vi "Update device interface.vi"(8 "error in (no error)":errorcluster, 10 "Found Instruments":string[][](array[string]), 11 "PIC-Device in":refnum<class "PIC-Device.lvclass">) -> (0 "error out":errorcluster, 3 "PIC-Device out":refnum<class "PIC-Device.lvclass">)   [LabVIEW 2020, in "PIC-Device.lvclass"]
uses:
  PIC-Device.lvclass
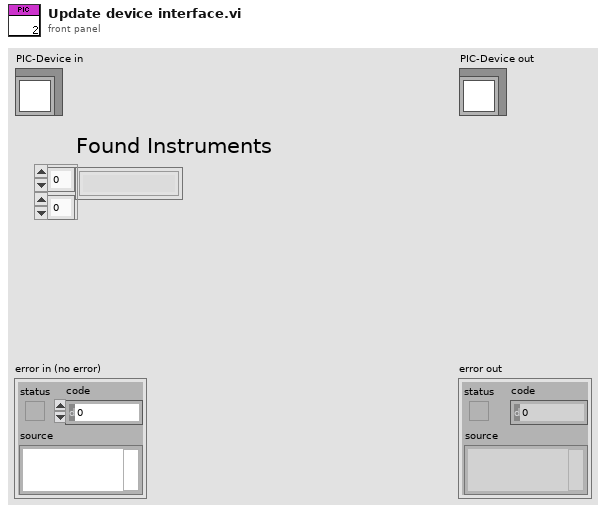
[diagram p1: front panel]
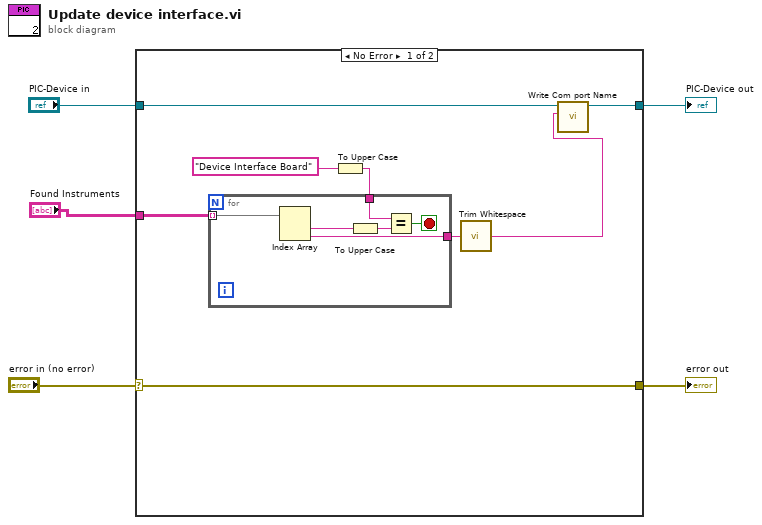
[diagram p0: block diagram]
diagram:
  n1 = case shown="No Error" "error in (no error)" {
    selector: "error in (no error)" -> [w13 w21]
    tunnel: [w13 w21] -> w4
    tunnel: [w11 w20] -> w3
    tunnel: "PIC-Device in" -> [w12 w20]
    tunnel: "Found Instruments" -> [w10 _]
    frame No Error {
      n2 = To Upper Case(1:"Device Interface Board") -> (0:w8:string)
      n3 = for {
        tunnel: w10 -> [w19] mode=indexing
        tunnel: w8 -> [w17]
        tunnel: [w15] -> w7
        stop <- w14 stop-if-true
        n4 = Index Array(array=w19) -> (element #1=w18:string, element #2=w15:string)  [unwired: 2 in]
        n5 = To Upper Case(1:w18) -> (0:w16:string)
        n6 = Equal?(x=w17, y=w16) -> (x = y?=w14:bool)
      }
      n7 = call <vilib>:"Trim Whitespace.vi"("string"=w7) -> ("trimmed string"=w6:string)  [unwired: 1 in]
      n8 = call-dynamic "Write Com port Name.vi"("Com port Name"=w6, "Device in"=w12) -> ("Device out"=w11:refnum<class "PIC-Device.lvclass">)  [unwired: 9 in]
    }
    frame Error {
    }
  }
  "error out" <- w4
  "PIC-Device out" <- w3
